vi "four_color_2D_AFM_synched.vi"() -> ()   [LabVIEW 2017]
uses:
  <vilib>/DAQmx/write.llb/DAQmx Write (Analog DBL 1Chan 1Samp).vi
  <vilib>/DAQmx/write.llb/DAQmx Write (Analog 2D DBL NChan NSamp).vi
  <vilib>/DAQmx/write.llb/DAQmx Write (Analog 1D DBL NChan 1Samp).vi
  <vilib>/DAQmx/create/channels.llb/DAQmx Create Channel (AO-Voltage-Basic).vi
  <vilib>/DAQmx/miscellaneous.llb/DAQmx Fill In Error Info.vi
  <vilib>/DAQmx/configure/timing.llb/DAQmx Timing (Sample Clock).vi
  <vilib>/DAQmx/configure/trigger.llb/DAQmx Start Trigger (Digital Edge).vi
  <resource>/objmgr/daqmx.rc
panel:
  in  "Listbox 3":i32(listbox)=3
  in  "Laser 4 (0-10v)":dbl=3.0
  in  "Listbox 4":i32(listbox)=3
  in  "ON Time(ms)":dbl=300.0
  in  "OFF Time(ms)":dbl=100.0
  in  "Laser 1 (0-10v)":dbl=3.0
  in  "Laser 2 (0-10v)":dbl=3.0
  in  "Listbox":i32(listbox)=1
  in  "Listbox 2":i32(listbox)=3
  out "Expected AFM Frequency (HZ)":dbl
  in  "Laser 3 (0-10v)":dbl=3.0
  in  "Combined Movement (v)\nEquation: X * X Multiplier + Y * Y Multiplier":dbl(slide) min=-10.0 max=10.0 step=0.01 scale=-10.0..10.0
  in  "X (v)":dbl(slide) min=-10.0 max=10.0 step=0.01 scale=-10.0..10.0
  in  "Y (v)":dbl(slide) min=-10.0 max=10.0 step=0.01 scale=-10.0..10.0
  in  "ETL3 (v) [4.76V allows light passing through unaltered]":dbl(slide)=4.76 min=-10.0 max=10.0 step=0.01 scale=-10.0..10.0
  out "Diopter":dbl
  out "Focal Distance (um)":dbl
  in  "Y multiplier":dbl=1.0
  in  "X multiplier":dbl=-1.0
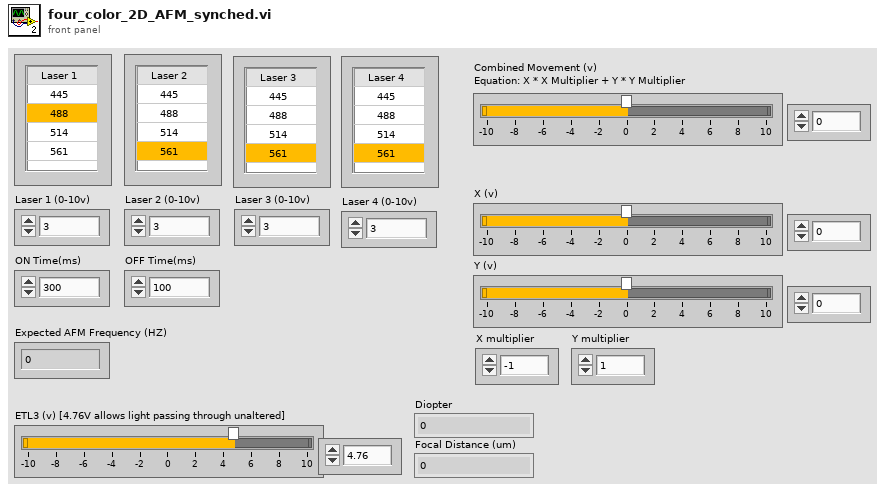
[diagram p1: front panel]
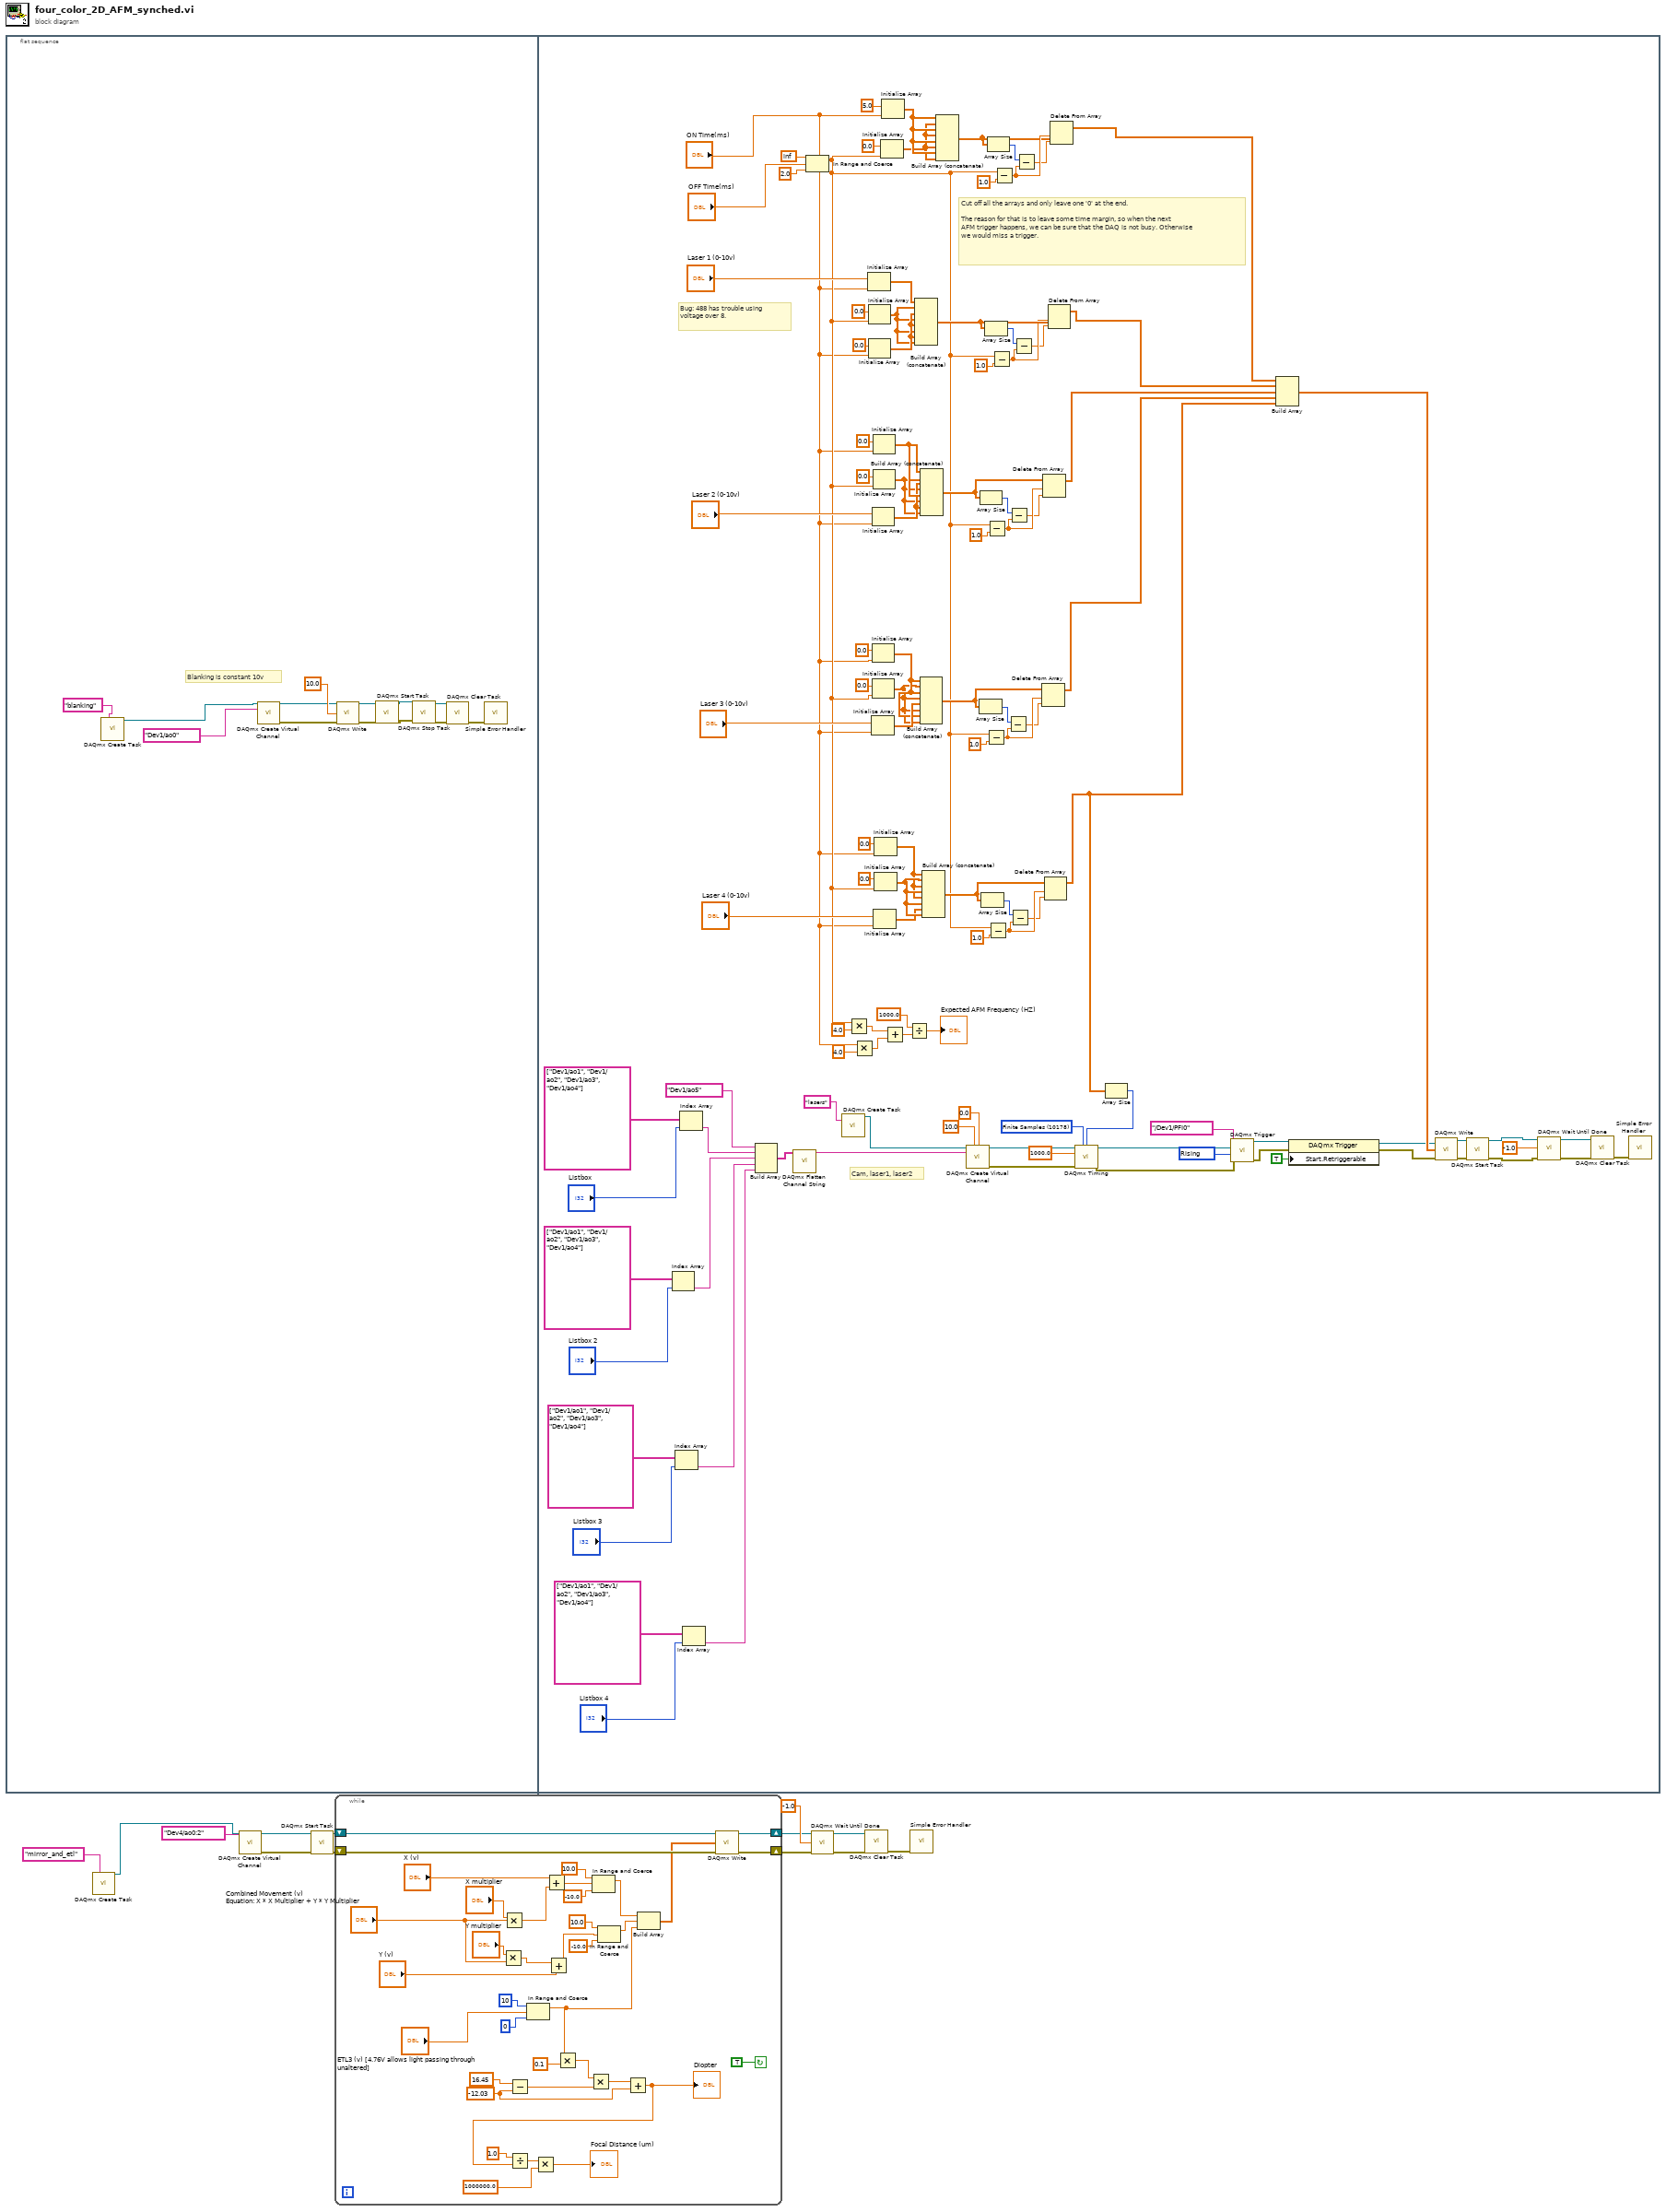
[diagram p0: block diagram]
diagram:
  n1 = flat-sequence {
    frame #0 {
      # "Blanking is constant 10v"
      n2 = call <vilib>:"DAQmx Create Task.vi"("new task name"="blanking" ("name to assign")) -> ("task out"=w16:refnum<k21>)  [unwired: 13 in, 1 out]
      n3 = call-poly <vilib>:"DAQmx Create Virtual Channel.vi"("task in"=w16, "physical channels"=tag "Dev1/ao0") -> ("task out"=w24:refnum<k21>, "error out"=w23:errorcluster)  [unwired: 12 in]
      n4 = call-poly <vilib>:"DAQmx Write.vi"("task/channels in"=w24, "data"=10.0, "error in"=w23) -> ("task out"=w22:refnum<k21>, "error out"=w21:errorcluster)  [unwired: 10 in, 1 out]
      n5 = call <vilib>:"DAQmx Start Task.vi"("task/channels in"=w22, "error in"=w21) -> ("task out"=w15:refnum<k21>, "error out"=w14:errorcluster)  [unwired: 12 in]
      n6 = call <vilib>:"DAQmx Stop Task.vi"("task/channels in"=w15, "error in"=w14) -> ("task out"=w20:refnum<k21>, "error out"=w19:errorcluster)  [unwired: 12 in]
      n7 = call <vilib>:"DAQmx Clear Task.vi"("task in"=w20, "error in"=w19) -> ("error out"=w26:errorcluster)  [unwired: 13 in]
      n8 = call <vilib>:"Simple Error Handler.vi"("error in (no error)"=w26) -> ()  [unwired: 4 in, 5 out]
    }
    frame #1 {
      w82 = 10280 items=["Rising"=10280, "Falling"=10171] ("edge")
      w78 = 10178 items=["Finite Samples"=10178, "Continuous Samples"=10123, "Hardware Timed Single Point"=12522] ("sample mode")
      # "Bug: 488 has trouble using voltage over 8."
      # "Cut off all the arrays and only leave one '0' at the end.\n\nThe reason for that is to leave some time margin, so when the next \nAFM trigger happens, we can be sure that the DAQ is not busy. Otherwise\nwe would miss a trigger."
      # "Cam, laser1, laser2"
      n9 = Index Array(array=tag[] ["Dev1/ao1", "Dev1/ao2", "Dev1/ao3", "Dev1/ao4"], index="Listbox 2") -> (element=w132:tag)
      n10 = Index Array(array=tag[] ["Dev1/ao1", "Dev1/ao2", "Dev1/ao3", "Dev1/ao4"], index="Listbox 3") -> (element=w64:tag)
      n11 = Index Array(array=tag[] ["Dev1/ao1", "Dev1/ao2", "Dev1/ao3", "Dev1/ao4"], index="Listbox") -> (element=w131:tag)
      n12 = Index Array(array=tag[] ["Dev1/ao1", "Dev1/ao2", "Dev1/ao3", "Dev1/ao4"], index="Listbox 4") -> (element=w27:tag)
      n13 = Build Array(tag "Dev1/ao5" ("physical channels"), w131, w132, w64, w27) -> (w133:tag[])
      n14 = call <vilib>:"DAQmx Flatten Channel String.vi"("names in"=w133) -> ("names out"=w136:string)  [unwired: 13 in, 1 out]
      n15 = In Range and Coerce(upper limit=inf, x="OFF Time(ms)", lower limit=2.0) -> (coerced(x)=w35:dbl)  [unwired: 1 out]
      n16 = call <vilib>:"DAQmx Create Task.vi"("new task name"="lasers" ("name to assign")) -> ("task out"=w138:refnum<k21>)  [unwired: 13 in, 1 out]
      n17 = Multiply(x=w35, y=4.0) -> (x*y=w121:dbl)
      n18 = Multiply(x="ON Time(ms)", y=4.0) -> (x*y=w120:dbl)
      n19 = Initialize Array("Laser 1 (0-10v)", "ON Time(ms)") -> (w96:dbl[])
      n20 = Initialize Array(0.0 ("element"), w35) -> (w49:dbl[])
      n21 = Initialize Array(0.0 ("element"), "ON Time(ms)") -> (w50:dbl[])
      n22 = Initialize Array("Laser 3 (0-10v)", "ON Time(ms)") -> (w53:dbl[])
      n23 = Initialize Array("Laser 2 (0-10v)", "ON Time(ms)") -> (w48:dbl[])
      n24 = Initialize Array(0.0 ("element"), "ON Time(ms)") -> (w46:dbl[])
      n25 = Initialize Array(0.0 ("element"), w35) -> (w45:dbl[])
      n26 = Initialize Array(0.0 ("element"), "ON Time(ms)") -> (w54:dbl[])
      n27 = Initialize Array(0.0 ("element"), w35) -> (w47:dbl[])
      n28 = Initialize Array("Laser 4 (0-10v)", "ON Time(ms)") -> (w32:dbl[])
      n29 = Initialize Array(0.0 ("element"), "ON Time(ms)") -> (w33:dbl[])
      n30 = Initialize Array(0.0 ("element"), w35) -> (w37:dbl[])
      n31 = Initialize Array(0.0 ("element"), w35) -> (w51:dbl[])
      n32 = Initialize Array(5.0 ("element"), "ON Time(ms)") -> (w52:dbl[])
      n33 = Add(x=w121, y=w120) -> (x+y=w122:dbl)
      n34 = Divide(x=1000.0, y=w122) -> (x/y=→"Expected AFM Frequency (HZ)":dbl)
      n35 = Build Array (concatenate)(w96, w49, w50, w49, w50, w49, w50, w49) -> (w100:dbl[])
      n36 = Build Array (concatenate)(w46, w45, w46, w45, w53, w45, w46, w45) -> (w63:dbl[])
      n37 = Build Array (concatenate)(w54, w47, w48, w47, w54, w47, w48, w47) -> (w104:dbl[])
      n38 = Build Array (concatenate)(w33, w37, w33, w37, w33, w37, w32, w37) -> (w44:dbl[])
      n39 = Build Array (concatenate)(w52, w51, w52, w51, w52, w51, w52, w51) -> (w92:dbl[])
      n40 = call-poly <vilib>:"DAQmx Create Virtual Channel.vi"("task in"=w138, "maximum value"=10.0, "minimum value"=0.0, "physical channels"=w136) -> ("task out"=w112:refnum<k21>, "error out"=w113:errorcluster)  [unwired: 10 in]
      n41 = Array Size(array=w63) -> (size(s)=w60:i32)
      n42 = Array Size(array=w104) -> (size(s)=w101:i32)
      n43 = Array Size(array=w44) -> (size(s)=w41:i32)
      n44 = Array Size(array=w100) -> (size(s)=w97:i32)
      n45 = Subtract(x=w35, y=1.0) -> (x-y=w62:dbl)
      n46 = Subtract(x=w35, y=1.0) -> (x-y=w103:dbl)
      n47 = Array Size(array=w92) -> (size(s)=w93:i32)
      n48 = Subtract(x=w35, y=1.0) -> (x-y=w43:dbl)
      n49 = Subtract(x=w35, y=1.0) -> (x-y=w99:dbl)
      n50 = Subtract(x=w35, y=1.0) -> (x-y=w95:dbl)
      n51 = Subtract(x=w60, y=w62) -> (x-y=w61:dbl)
      n52 = Subtract(x=w101, y=w103) -> (x-y=w102:dbl)
      n53 = Subtract(x=w41, y=w43) -> (x-y=w42:dbl)
      n54 = Subtract(x=w97, y=w99) -> (x-y=w98:dbl)
      n55 = Subtract(x=w93, y=w95) -> (x-y=w94:dbl)
      n56 = Delete From Array(array=w63, length=w62, index=w61) -> (array with subset deleted=w55:dbl[])  [unwired: 1 out]
      n57 = Delete From Array(array=w104, length=w103, index=w102) -> (array with subset deleted=w126:dbl[])  [unwired: 1 out]
      n58 = Delete From Array(array=w44, length=w43, index=w42) -> (array with subset deleted=w31:dbl[])  [unwired: 1 out]
      n59 = Delete From Array(array=w100, length=w99, index=w98) -> (array with subset deleted=w124:dbl[])  [unwired: 1 out]
      n60 = Delete From Array(array=w92, length=w95, index=w94) -> (array with subset deleted=w123:dbl[])  [unwired: 1 out]
      n61 = Array Size(array=w31) -> (size(s)=w137:i32)
      n62 = call-poly <vilib>:"DAQmx Timing.vi"("task/channels in"=w112, "sample mode"=w78, "samples per channel"=w137, "rate"=1000.0, "error in"=w113) -> ("task out"=w114:refnum<k21>, "error out"=w115:errorcluster)  [unwired: 9 in]
      n63 = call-poly <vilib>:"DAQmx Trigger.vi"("task/channels in"=w114, "source"=tag "/Dev1/PFI0", "edge"=w82, "error in"=w115) -> ("task out"=w116:refnum<k21>, "error out"=w119:errorcluster)  [unwired: 10 in]
      n64 = Build Array(w123, w124, w126, w55, w31) -> (w125:dbl[][])
      n65 = property class="DAQmx Trigger"(reference=w116, error in=w119, "Start.Retriggerable"=TRUE) -> (reference out=w117:refnum<k21>, error out=w118:errorcluster)
      n66 = call-poly <vilib>:"DAQmx Write.vi"("task/channels in"=w117, "data"=w125, "error in"=w118) -> ("task out"=w110:refnum<k21>, "error out"=w111:errorcluster)  [unwired: 10 in, 1 out]
      n67 = call <vilib>:"DAQmx Start Task.vi"("task/channels in"=w110, "error in"=w111) -> ("task out"=w109:refnum<k21>, "error out"=w108:errorcluster)  [unwired: 12 in]
      n68 = call <vilib>:"DAQmx Wait Until Done.vi"("task/channels in"=w109, "timeout (sec)"=-1.0, "error in"=w108) -> ("task out"=w106:refnum<k21>, "error out"=w107:errorcluster)  [unwired: 11 in]
      n69 = call <vilib>:"DAQmx Clear Task.vi"("task in"=w106, "error in"=w107) -> ("error out"=w105:errorcluster)  [unwired: 13 in]
      n70 = call <vilib>:"Simple Error Handler.vi"("error in (no error)"=w105) -> ()  [unwired: 4 in, 5 out]
    }
  }
  n71 = call <vilib>:"DAQmx Create Task.vi"("new task name"="mirror_and_etl" ("name to assign")) -> ("task out"=w1:refnum<k21>)  [unwired: 13 in, 1 out]
  n72 = call-poly <vilib>:"DAQmx Create Virtual Channel.vi"("task in"=w1, "physical channels"=tag "Dev4/ao0:2") -> ("task out"=w6:refnum<k21>, "error out"=w5:errorcluster)  [unwired: 12 in]
  n73 = call <vilib>:"DAQmx Start Task.vi"("task/channels in"=w6, "error in"=w5) -> ("task out"=w8:refnum<k21>, "error out"=w7:errorcluster)  [unwired: 12 in]
  n74 = while {
    shift-right: [w172] -> w3
    shift-left: w8 -> [w174]
    shift-right: [w171] -> w4
    shift-left: w7 -> [w173]
    stop <- TRUE continue-if-true
    w148 = -12.03 ("x")
    n75 = Multiply(x="Y multiplier", y="Combined Movement (v)\nEquation: X * X Multiplier + Y * Y Multiplier") -> (x*y=w159:dbl)
    n76 = Multiply(x="X multiplier", y="Combined Movement (v)\nEquation: X * X Multiplier + Y * Y Multiplier") -> (x*y=w168:dbl)
    n77 = Subtract(x=16.45 ("y"), y=w148) -> (x-y=w150:dbl)
    n78 = In Range and Coerce(upper limit=10, x="ETL3 (v) [4.76V allows light passing through unaltered]", lower limit=0) -> (coerced(x)=w147:dbl)  [unwired: 1 out]
    n79 = Add(x="X (v)", y=w168) -> (x+y=w167:dbl)
    n80 = Add(x=w159, y="Y (v)") -> (x+y=w161:dbl)
    n81 = Multiply(x=w147, y=0.1) -> (x*y=w151:dbl)
    n82 = Multiply(x=w151, y=w150) -> (x*y=w149:dbl)
    n83 = In Range and Coerce(upper limit=10.0, x=w167, lower limit=-10.0) -> (coerced(x)=w164:dbl)  [unwired: 1 out]
    n84 = In Range and Coerce(upper limit=10.0, x=w161, lower limit=-10.0) -> (coerced(x)=w160:dbl)  [unwired: 1 out]
    n85 = Add(x=w149, y=w148) -> (x+y=w142:dbl)
    "Diopter" <- w142
    n86 = Divide(x=1.0, y=w142) -> (x/y=w157:dbl)
    n87 = Multiply(x=w157, y=1000000.0) -> (x*y=→"Focal Distance (um)":dbl)
    n88 = Build Array(w164, w160, w147) -> (w170:dbl[])
    n89 = call-poly <vilib>:"DAQmx Write.vi"("task/channels in"=w174, "data"=w170, "error in"=w173) -> ("task out"=w172:refnum<k21>, "error out"=w171:errorcluster)  [unwired: 10 in, 1 out]
  }
  n90 = call <vilib>:"DAQmx Wait Until Done.vi"("task/channels in"=w3, "timeout (sec)"=-1.0, "error in"=w4) -> ("task out"=w12:refnum<k21>, "error out"=w11:errorcluster)  [unwired: 11 in]
  n91 = call <vilib>:"DAQmx Clear Task.vi"("task in"=w12, "error in"=w11) -> ("error out"=w13:errorcluster)  [unwired: 13 in]
  n92 = call <vilib>:"Simple Error Handler.vi"("error in (no error)"=w13) -> ()  [unwired: 4 in, 5 out]
